vi "CALC_MARK_TARG.vi"(0 "VISA IN":refnum<visa-resource-name>, 1 "Marker number":i32, 2 "Target Value":dbl format="%_5g", 5 "error in":errorcluster, 7 "Channel":i32) -> (14 "VISA Out":refnum<visa-resource-name>, 19 "error out":errorcluster)   [LabVIEW 2018, in "PNA-X.lvlib"]
doc: "CALCulate<cnum>:MARKer<mkr>:TARGet <num> \n(Read-Write) Sets the target value for the specified marker when doing Target Searches with \nCALC:MARK:FUNC:SEL <TARGet | RTARget | LTARget> \nSee Critical Note \nParameters \n<cnum> Channel number of the measurement. There must be a selected measurement \non that channel. If unspecified, <cnum> is set to 1. \n<mkr> Any marker number from 1 to 10; if unspecified, value is set to 1. \n<num> Target value to search for; Units are NOT allowed. \nExamples CALC:MARK:TARG 2.5 \ncalculate2:marker8:target -10.3 \nQuery Syntax CALCulate<cnum>:MARKer<mkr>:TARGet? \nReturn Type Numeric \nDefault 0"
uses:
  PNA-X.lvlib
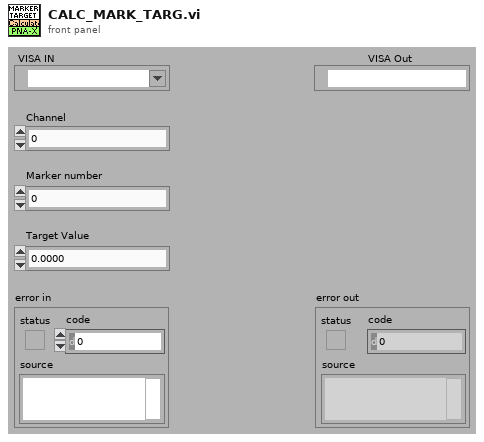
[diagram p1: front panel]
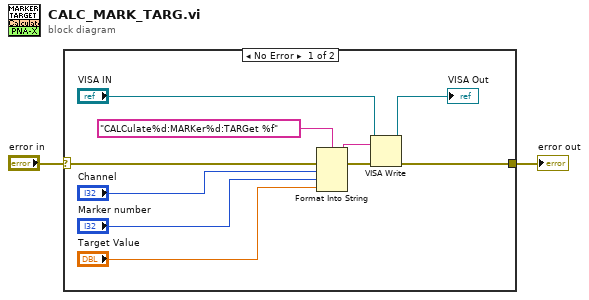
[diagram p0: block diagram]
diagram:
  n1 = case shown="No Error" "error in" {
    selector: "error in" -> [w12 w13]
    tunnel: [w7 w13] -> w1
    frame No Error {
      n2 = Format Into String(format string="CALCulate%d:MARKer%d:TARGet %f" ("Cmdline"), error in=w12, "Channel", "Marker number", "Target Value") -> (resulting string=w10:string, error out=w11:errorcluster)  [unwired: 1 in]
      n3 = VISA Write(VISA resource name="VISA IN", write buffer=w10, error in (no error)=w11) -> (VISA resource name out=→"VISA Out":refnum<visa-resource-name>, error out=w7:errorcluster)  [unwired: 1 out]
    }
    frame Error {
    }
  }
  "error out" <- w1
